vi "Global 1.vi"() -> ()   [LabVIEW 2020, in "NetAn.lvclass"]
uses:
  Proto/NetAn.lvclass
panel:
  in  "Largest":i32=-1
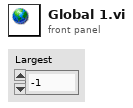
[diagram p1: front panel]
diagram:
